vi "MainPane Slide.vi"(8 "error in (no error)":errorcluster, 9 "Slide Direction":T1=enum."Back", 10 "Enqueuer":refnum<class "Message Enqueuer.lvclass">, 11 "DemoMain in":refnum<class "DemoMain.lvclass">) -> (0 "error out":errorcluster, 3 "DemoMain out":refnum<class "DemoMain.lvclass">)   [LabVIEW 2012, in "Win8uiDemo.lvlib" / "DemoMain.lvclass"]
uses:
  DemoMain.lvclass
  <vilib>/ActorFramework/Message Enqueuer/Message Enqueuer.lvclass
  Win8uiFramework/Slide Direction.ctl
  DemoMain.lvclass/DemoMain.ctl
  Win8uiFramework/MainController.lvclass/MainController.ctl
  Win8uiFramework/MainController.lvclass
  Win8uiFramework/Write MainPane Enqueuer.vi
  Read GridView Enqueuer.vi
  Win8uiFramework/Win8uiFramework.lvlib
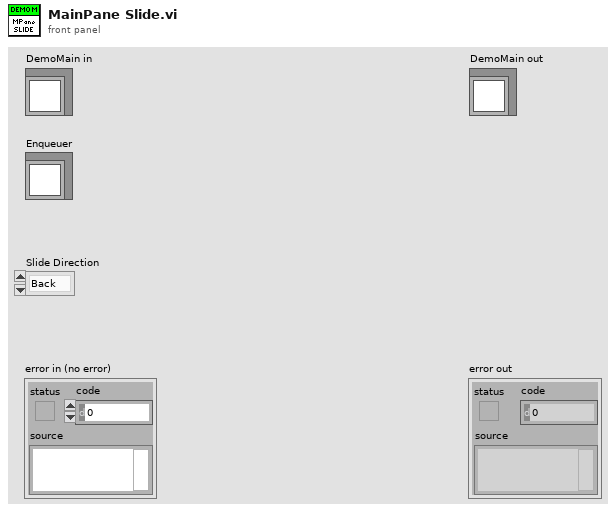
[diagram p1: front panel]
types:
  T1 = typedef "Win8uiFramework.lvlib/Slide Direction.ctl" = enum16{"Forwards", "Back"}
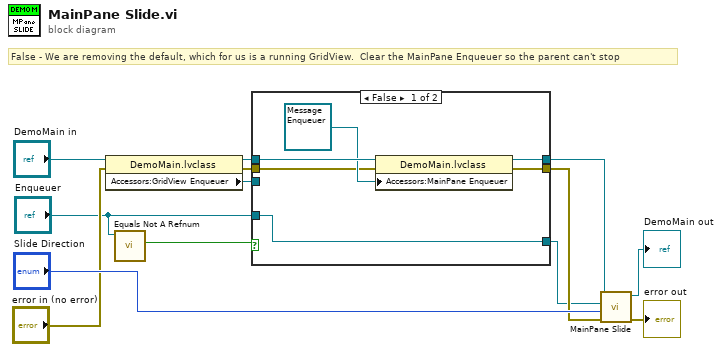
[diagram p0: block diagram]
diagram:
  # "False - We are removing the default, which for us is a running GridView.  Clear the MainPane Enqueuer so the parent can't stop"
  n1 = property class="DemoMain.lvclass"(reference="DemoMain in", error in="error in (no error)") -> (reference out=w8:refnum<class "DemoMain.lvclass">, error out=w7:errorcluster, "Accessors:GridView Enqueuer"=w4:refnum<class "Message Enqueuer.lvclass">)
  n2 = call <vilib>:"Equals Not A Refnum.vi"("Message Enqueuer"="Enqueuer") -> ("Not a refnum?"=w6:bool)  [unwired: 10 in]
  n3 = case shown="False" w6 {
    tunnel: w8 -> [w19 w22]
    tunnel: w7 -> [w15 w21]
    tunnel: "Enqueuer" -> [w14 _]
    tunnel: w4 -> [_ w20]
    tunnel: [w14 w20] -> w1
    tunnel: [w18 w22] -> w3
    tunnel: [w17 w21] -> w2
    frame False {
      n4 = property class="DemoMain.lvclass"(reference=w19, error in=w15, "Accessors:MainPane Enqueuer"=refnum<class "Message Enqueuer.lvclass"> refnum ("MainPane Enqueuer")) -> (reference out=w18:refnum<class "DemoMain.lvclass">, error out=w17:errorcluster)
    }
    frame True {
    }
  }
  n5 = call-parent "MainPane Slide.vi"("error in (no error)"=w2, "Slide Direction"="Slide Direction", "Enqueuer"=w1, "MainController in"=w3) -> ("error out"=→"error out":errorcluster, "MainController out"=→"DemoMain out":refnum<class "DemoMain.lvclass">)  [unwired: 6 in]
